vi "Get json data array.vi"(8 "error in (no error)":errorcluster, 11 "Json data string":string) -> (0 "error out":errorcluster, 2 "data items":i32, 3 "Json data array":string[](array[string]))   [LabVIEW 2013]
panel:
  out "IDs":i32
  out "Json ID array":string[](array[string])
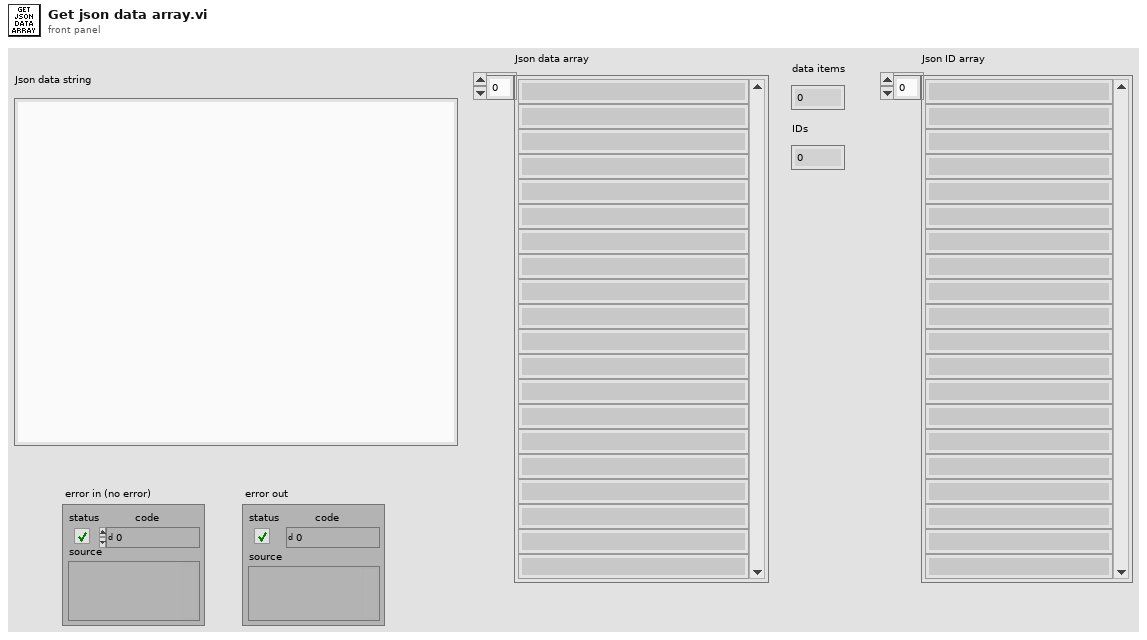
[diagram p1: front panel]
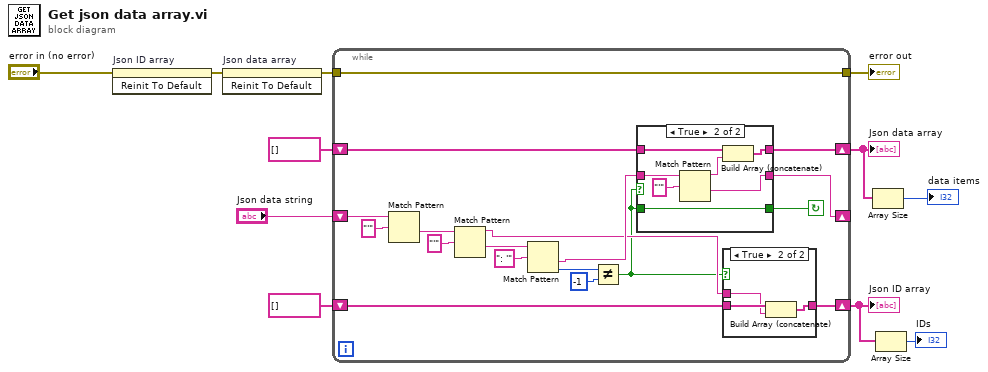
[diagram p0: block diagram]
diagram:
  n1 = invoke on="Json ID array" class="Arr (strict)" method="Reinit To Default"(error in="error in (no error)") -> (error out=w3:errorcluster)  [unwired: 2 in, 2 out]
  n2 = invoke on="Json data array" class="Arr (strict)" method="Reinit To Default"(error in=w3) -> (error out=w7:errorcluster)  [unwired: 2 in, 2 out]
  n3 = while {
    shift-right: [w22] -> _
    shift-left: "Json data string" -> [w19]
    shift-right: [w24] -> w9
    shift-left: string[] [] -> [w25]
    tunnel: w7 -> [w21]
    tunnel: [w21] -> w6
    shift-right: [w14] -> w2
    shift-left: string[] [] -> [w16]
    stop <- w23 continue-if-true
    n4 = Match Pattern(string=w19, regular expression="'") -> (after substring=w17:string)  [unwired: 1 in, 3 out]
    n5 = Match Pattern(string=w17, regular expression="'") -> (before substring=w15:string, after substring=w13:string)  [unwired: 1 in, 2 out]
    n6 = Match Pattern(string=w13, regular expression=": '") -> (after substring=w28:string, offset past match=w27:i32)  [unwired: 1 in, 2 out]
    n7 = Not Equal?(x=w27, y=-1) -> (x != y?=w12:bool)
    n8 = case shown="True" w12 {
      selector: w12 -> [w34 _]
      tunnel: w28 -> [w35 w40]
      tunnel: w25 -> [w36 w43]
      tunnel: [w36 w42] -> w24
      tunnel: [w34 w39] -> w23
      tunnel: [w35 w41] -> w22
      tunnel: w12 -> [_ w39]
      frame False {
      }
      frame True {
        n9 = Match Pattern(string=w40, regular expression="'") -> (before substring=w37:string, after substring=w41:string)  [unwired: 1 in, 2 out]
        n10 = Build Array (concatenate)(w43, w37) -> (w42:string[])
      }
    }
    n11 = case shown="True" w12 {
      tunnel: w16 -> [w30 w33]
      tunnel: w15 -> [_ w32]
      tunnel: [w30 w31] -> w14
      frame False {
      }
      frame True {
        n12 = Build Array (concatenate)(w33, w32) -> (w31:string[])
      }
    }
  }
  "error out" <- w6
  "Json data array" <- w9
  "Json ID array" <- w2
  n13 = Array Size(array=w9) -> (size(s)=→"data items":i32)
  n14 = Array Size(array=w2) -> (size(s)=→"IDs":i32)
